vi "Auto_Routine_StraightTwoPieceTRAJ.vi"(8 "error in (no error)":errorcluster) -> (0 "error out":errorcluster)   [LabVIEW 2023]
doc: "Moves from middle of the speaker to the middle note on robot starting line and back \n*****DOES NOT HAVE WAIT AFTER COMPLETE*****\n-Sets arm to speaker Pose\n-Pre rev\n-Waits for arm (to get to speaker shooot pose)\n-Shoots note\n-Waits for box to shoot note\n-Sets arm to floor\n-Runs intake\n-Moves to note\n-Sets arm to speaker pose\n-20 ms wait\n-Goes back to speaker (while waiting for note to intake and pre rev-ing)\n-Waits for arm (to be at speaker shoot pose)\n-Shoots note\n-Waits for shoot to be done \n-Sets arm to floor"
uses:
  Trajectory/TrajectoryGlobals.vi
  <vilib>/Rock Robotics/WPI/ThirdParty/JAS_Junk/TrajLib/Trajectory_Library.lvlib
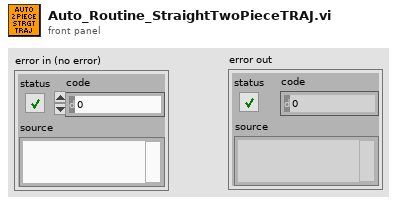
[diagram p1: front panel]
types:
  T1 = typedef "Trajectory_Library.lvlib/TRAJECTORY.ctl" = cluster{"TotalTImeSecs":dbl, "States":T2[]}
  T2 = typedef "Trajectory_Library.lvlib/TRAJ_STATE.ctl" = cluster{"TimeSeconds":dbl, "Velocity":dbl, "Acceleration":dbl, "POSE":T3, "Curvature":dbl}
  T3 = typedef "Trajectory_Library.lvlib/POSE2D.ctl" = cluster{"TRANSLATION":T4, "ROTATION":T5}
  T4 = typedef "Trajectory_Library.lvlib/TRANSLATION2D.ctl" = cluster{"X":dbl, "Y":dbl}
  T5 = typedef "Trajectory_Library.lvlib/ROTATION2D.ctl" = cluster{"VALUE":dbl, "COS":dbl, "SIN":dbl}
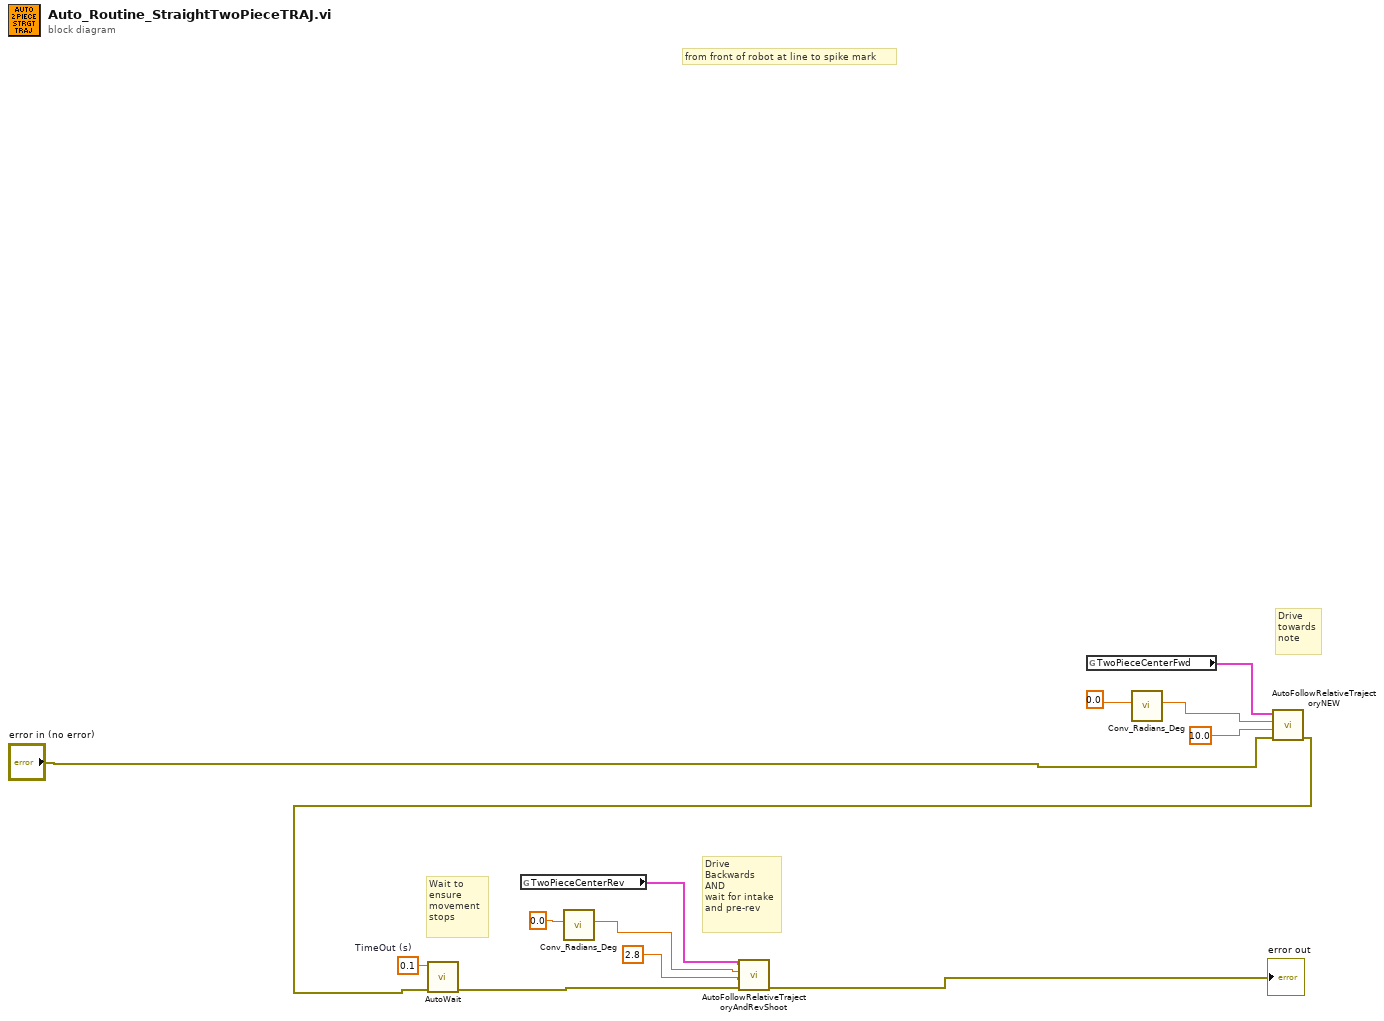
[diagram p0: block diagram]
diagram:
  w4 = 0.1  # TimeOut (s)
  # "Wait to\nensure \nmovement\nstops"
  # "Drive\nBackwards\nAND\nwait for intake\nand pre-rev"
  # "Drive\ntowards\nnote"
  # "from front of robot at line to spike mark"
  n1 = global read "TrajectoryGlobals.vi" "TwoPieceCenterRev"() -> (w8:T1)
  n2 = call <vilib>:"Conv_Radians_Deg.vi"("Radians"=0.0) -> ("Degrees"=w7:dbl)  [unwired: 10 in]
  n3 = global read "TrajectoryGlobals.vi" "TwoPieceCenterFwd"() -> (w13:T1)
  n4 = call <vilib>:"Conv_Radians_Deg.vi"("Radians"=0.0) -> ("Degrees"=w11:dbl)  [unwired: 10 in]
  n5 = call "AutoFollowRelativeTrajectoryNEW.vi"("error in (no error)"="error in (no error)", "TimeOut (s)"=10.0, "End Orientation"=w11, "Trajectory"=w13) -> ("error out"=w3:errorcluster)  [unwired: 7 in]
  n6 = call "AutoWait.vi"("error in (no error)"=w3, "TimeOut (s)"=w4) -> ("error out"=w5:errorcluster)  [unwired: 9 in]
  n7 = call "AutoFollowRelativeTrajectoryAndRevShoot.vi"("error in (no error)"=w5, "TimeOut (s)"=2.8, "End Orientation"=w7, "Trajectory"=w8) -> ("error out"=→"error out":errorcluster)  [unwired: 7 in]
